vi "Change SP.vi"(1 "error in":errorcluster, 2 "Set Point":u32, 3 "Adress":u8 format="%x", 4 "VISA resource name":refnum<visa-resource-name>="ASRL2::INSTR") -> (0 "error out":errorcluster)   [LabVIEW 2009]
uses:
  <vilib>/Instr/_visa.llb/VISA Configure Serial Port (Instr).vi
panel:
  out "Write buffer":string
  out "Serial Settings:Number of Bytes at Serial Port":u32
  out "unsigned byte array":u8[](array[numeric]) format="%x"
  out "Read buffer":string
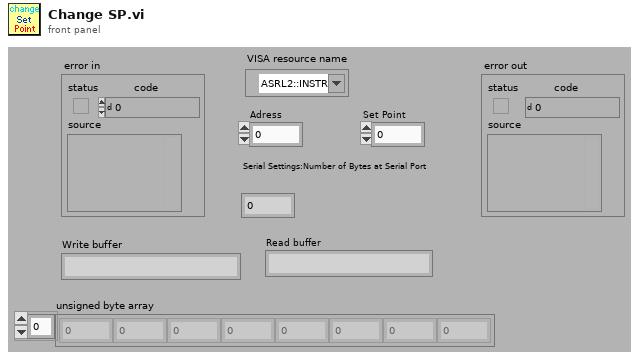
[diagram p1: front panel]
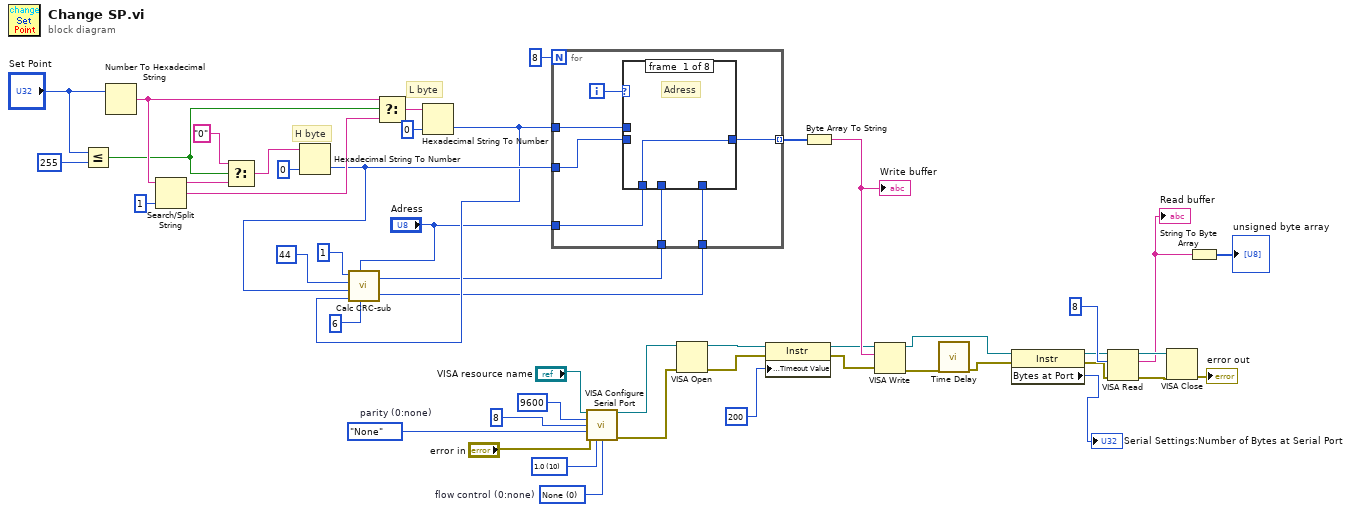
[diagram p0: block diagram]
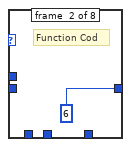
[diagram p2: hidden frame]
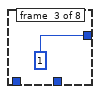
[diagram p3: hidden frame]
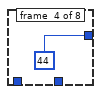
[diagram p4: hidden frame]
diagram:
  w9 = enum16{"None", "Odd", "Even", "Mark", "Space"}."None"  # parity (0:none)
  w5 = u16 0 items=["None"=0, "XON/XOFF"=1, "RTS/CTS"=2, "DTR/DSR"=4]  # flow control (0:none)
  w6 = u16 10 items=["1.0"=10, "1.5"=15, "2.0"=20] ("stop bits (10: 1 bit)")
  # "L byte"
  # "H byte"
  n1 = Less Or Equal?(x="Set Point", y=u32 255) -> (x <= y?=w26:bool)
  n2 = Number To Hexadecimal String(2:"Set Point") -> (0:w32:string)  [unwired: 1 out]
  n3 = Search/Split String(string=w32, offset (0)=1) -> (substring before match=w31:string, match + rest of string=w29:string)  [unwired: 2 out]
  n4 = Select(t="0", s=w26, f=w31) -> (s? t:f=w27:string)
  n5 = Hexadecimal String To Number(string=w27, default (0uL)=u8 0 ("default (0 U32)")) -> (number=w21:u8)  [unwired: 2 out]
  n6 = Select(t=w32, s=w26, f=w29) -> (s? t:f=w28:string)
  n7 = Hexadecimal String To Number(string=w28, default (0uL)=u8 0 ("default (0 U32)")) -> (number=w20:u8)  [unwired: 2 out]
  n8 = call "Calc CRC-sub.vi"("Command"=u8 6, "Adress"="Adress", "Data L"=w20, "Data H"=w21, "Reg L"=u8 44 ("Reg-L"), "Reg H"=u8 1 ("Reg-H")) -> ("L byte"=w19:u8, "H byte"=w18:u8)
  n9 = for {
    N: 8 -> [_]
    tunnel: [w55] -> w49 mode=indexing
    tunnel: w21 -> [w54]
    tunnel: w20 -> [w53]
    tunnel: w19 -> [w52]
    tunnel: w18 -> [w51]
    tunnel: "Adress" -> [w50]
    i -> [w56]
    n10 = case shown="3" w56 {
      tunnel: [w57 u8 6 ("Command") u8 1 ("Reg-H") u8 44 ("Reg-L") w61 w62 w63 w64] -> w55
      tunnel: w54 -> [_ _ _ _ w61 _ _ _]
      tunnel: w53 -> [_ _ _ _ _ w62 _ _]
      tunnel: w52 -> [_ _ _ _ _ _ w63 _]
      tunnel: w51 -> [_ _ _ _ _ _ _ w64]
      tunnel: w50 -> [w57 _ _ _ _ _ _ _]
      frame #0 {
        # "Adress"
      }
      frame #1 {
        # "Function Cod"
      }
      frame #2 {
      }
      frame #3 {
      }
      frame #4 {
        # "Data H"
      }
      frame #5 {
        # "Data L"
      }
      frame #6 {
        # "CRC-L"
      }
      frame #7 {
        # "CRC-H"
      }
    }
  }
  n11 = call-poly "VISA Configure Serial Port"("VISA resource name"="VISA resource name", "baud rate (9600)"=u32 9600, "data bits (8)"=u16 8, "parity (0:none)"=w9, "error in (no error)"="error in", "stop bits (10: 1 bit)"=w6, "flow control (0:none)"=w5) -> ("VISA resource name out"=w2:refnum<visa-resource-name>, "error out"=w1:errorcluster)  [unwired: 7 out]
  n12 = VISA Open(error in (no error)=w1, VISA resource name=w2) -> (VISA resource name=w44:refnum<visa-resource-name>, error out=w43:errorcluster)  [unwired: 3 out]
  n13 = property class="Instr"(reference=w44, error in=w43, "General Settings:Timeout Value"=u32 200) -> (reference out=w42:refnum<visa-resource-name>, error out=w41:errorcluster)
  n14 = Byte Array To String(unsigned byte array=w49) -> (string=w46:string)
  "Write buffer" <- w46
  n15 = VISA Write(VISA resource name=w42, write buffer=w46, error in (no error)=w41) -> (VISA resource name out=w13:refnum<visa-resource-name>, error out=w12:errorcluster)  [unwired: 1 out]
  n16 = call "Time Delay"("error in (no error)"=w12) -> ("error out"=w11:errorcluster)  [unwired: 1 in, 9 out]
  n17 = property class="Instr"(reference=w13, error in=w11) -> (reference out=w37:refnum<visa-resource-name>, error out=w10:errorcluster, "Bytes at Port"=→"Serial Settings:Number of Bytes at Serial Port":u32)
  n18 = VISA Read(VISA resource name=w37, byte count=u32 8 ("byte count (0)"), error in (no error)=w10) -> (VISA resource name out=w40:refnum<visa-resource-name>, read buffer=w36:string, error out=w39:errorcluster)  [unwired: 1 out]
  "Read buffer" <- w36
  n19 = VISA Close(VISA resource name=w40, error in (no error)=w39) -> (error out=→"error out":errorcluster)
  n20 = String To Byte Array(string=w36) -> (unsigned byte array=→"unsigned byte array":u8[])
